vi "New Secure WebSocket Client.vi"(6 "server certificate validation":enum32{"Any Trusted CA", "None"}(ring), 7 "immutable TLS Configuration":refnum<k36>, 8 "error in (no error)":errorcluster, 9 "Timeout (5000ms)":i32=5000, 11 "WebSocket URL":string="wss://localhost:7123") -> (0 "error out":errorcluster, 3 "Secure WebSockets Client out":refnum<class "Secure WebSockets Client.lvclass">)   [LabVIEW 2020, in "Secure WebSockets Client.lvclass"]
doc: "Creates a new WebSockets Client connection, using SSL/TLS if a Secure WebSockets URL (wss://) is specified."
uses:
  Secure WebSockets Client.lvclass
  C:/Program Files (x86)/National Instruments/LabVIEW 2020/vi.lib/MediaMongrels Ltd/WebSockets/WebSockets/WebSocket/WebSocket.lvclass
  C:/Program Files (x86)/National Instruments/LabVIEW 2020/vi.lib/MediaMongrels Ltd/WebSockets/WebSockets/WebSocket Client/WebSocket Client.lvclass
  <vilib>/MediaMongrels Ltd/WebSockets/Sockets/VISA TCP Socket/VISA TCP.lvclass
  C:/Program Files (x86)/National Instruments/LabVIEW 2020/vi.lib/MediaMongrels Ltd/WebSockets/Sockets/Socket/Socket.lvclass
  <vilib>/MediaMongrels Ltd/WebSockets/WebSockets/WebSocket/WebSocket.lvclass/WebSocket.ctl
  <vilib>/MediaMongrels Ltd/WebSockets/WebSockets/WebSocket Client/WebSocket Client.lvclass/WebSocket Client.ctl
  <vilib>/MediaMongrels Ltd/WebSockets/WebSockets/WebSocket/Write Socket.vi
  <vilib>/MediaMongrels Ltd/WebSockets/WebSockets/WebSocket Client/Write URL.vi
  <vilib>/MediaMongrels Ltd/WebSockets/WebSockets/WebSocket/WebSocket.lvclass
  <vilib>/MediaMongrels Ltd/WebSockets/WebSockets/WebSocket Client/WebSocket Client.lvclass
  Secure Sockets Addon/Secure Sockets Addon.lvlib
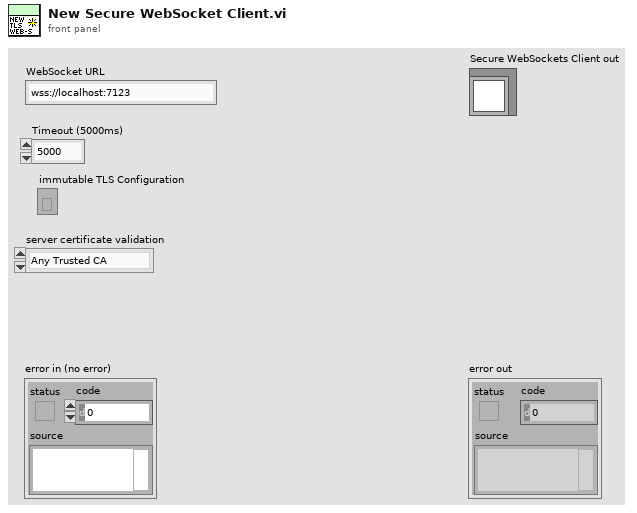
[diagram p1: front panel]
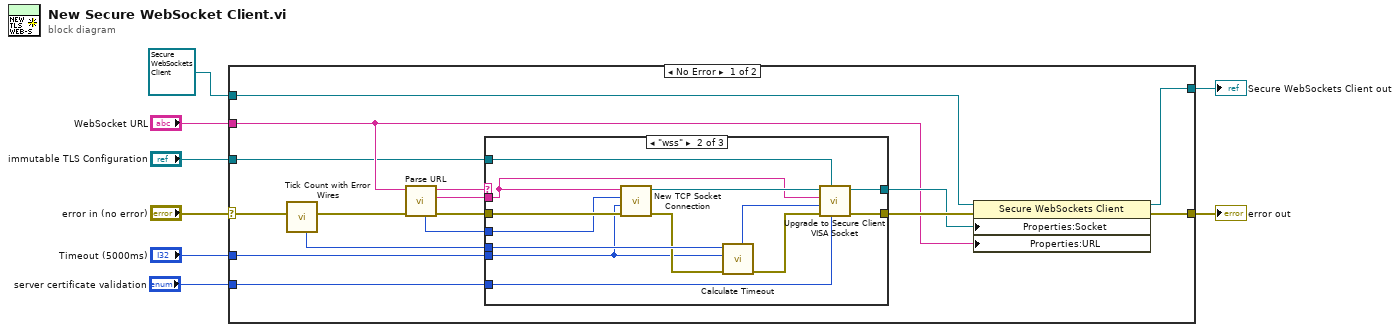
[diagram p0: block diagram]
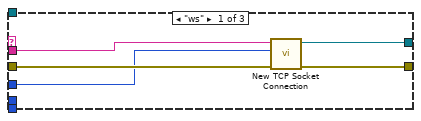
[diagram p2: hidden frame]
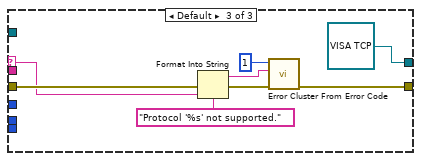
[diagram p3: hidden frame]
diagram:
  n1 = case shown="No Error" "error in (no error)" {
    selector: "error in (no error)" -> [w19 w51]
    tunnel: [w23 w51] -> w7
    tunnel: [w20 w50] -> w6
    tunnel: "WebSocket URL" -> [w15 _]
    tunnel: "Timeout (5000ms)" -> [w18 _]
    tunnel: refnum<class "Secure WebSockets Client.lvclass"> refnum ("Secure WebSockets Client.lvclass") -> [w22 w50]
    tunnel: "server certificate validation" -> [w10 _]
    tunnel: "immutable TLS Configuration" -> [w9 _]
    frame No Error {
      n2 = call <vilib>:"Tick Count with Error Wires.vi"("error in (no error)"=w19) -> ("error out"=w11:errorcluster, "millisecond timer value"=w17:u32)  [unwired: 9 in]
      n3 = call <vilib>:"Parse URL.vi"("error in (no error)"=w11, "WebSocket URL"=w15) -> ("error out"=w16:errorcluster, "host"=w13:string, "protocol"=w14:string, "port"=w12:u16)  [unwired: 5 in, 1 out]
      n4 = case shown="\"wss\"" w14 {
        selector: w14 -> [_ _ w44]
        tunnel: w16 -> [w27 w39 w48]
        tunnel: [w27 w33 w49] -> w24
        tunnel: [w26 w34 refnum<class "VISA TCP.lvclass"> refnum ("VISA TCP out")] -> w21
        tunnel: w18 -> [_ w36 _]
        tunnel: w17 -> [_ w40 _]
        tunnel: w13 -> [w28 w32 _]
        tunnel: w12 -> [w25 w38 _]
        tunnel: w10 -> [_ w30 _]
        tunnel: w9 -> [_ w29 _]
        frame "ws" {
          n5 = call <vilib>:"New TCP Socket Connection.vi"("error in (no error)"=w27, "Port"=w25, "Hostname / IP"=w28) -> ("VISA TCP out"=w26:refnum<class "VISA TCP.lvclass">)  [unwired: 7 in, 1 out]
        }
        frame "wss" {
          n6 = call <vilib>:"New TCP Socket Connection.vi"("error in (no error)"=w39, "timeout ms (5000)"=w36, "Port"=w38, "Hostname / IP"=w32) -> ("error out"=w37:errorcluster, "VISA TCP out"=w35:refnum<class "VISA TCP.lvclass">)  [unwired: 6 in]
          n7 = call <vilib>:"Calculate Timeout.vi"("error in (no error)"=w37, "timeout ms"=w36, "t0"=w40) -> ("error out"=w41:errorcluster, "new timeout ms"=w31:i32)  [unwired: 6 in, 1 out]
          n8 = call "Upgrade to Secure Client VISA Socket.vi"("server certificate validation"=w30, "immutable TLS Configuration"=w29, "error in (no error)"=w41, "timeout (5000ms)"=w31, "Server Hostname"=w32, "VISA TCP Socket in"=w35) -> ("error out"=w33:errorcluster, "Secure VISA TCP Socket out"=w34:refnum<class "VISA TCP.lvclass">)  [unwired: 3 in, 1 out]
        }
        frame Default {
          n9 = Format Into String(format string="Protocol '%s' not supported.", error in=w48, w44) -> (resulting string=w46:string, error out=w47:errorcluster)  [unwired: 1 in]
          n10 = call <vilib>:"Error Cluster From Error Code.vi"("error in (no error)"=w47, "error message (\"\")"=w46, "error code (0)"=1) -> ("error out"=w49:errorcluster)  [unwired: 6 in]
        }
      }
      n11 = property class="Secure WebSockets Client"(reference=w22, error in=w24, "Properties:Socket"=w21, "Properties:URL"=w15) -> (reference out=w20:refnum<class "Secure WebSockets Client.lvclass">, error out=w23:errorcluster)
    }
    frame Error {
    }
  }
  "error out" <- w7
  "Secure WebSockets Client out" <- w6
